vi "CRC32-CITT.vi"(8 "error in (no error)":errorcluster caption="错误输入（无错误）", 11 "Data":u8[](array[numeric]) format="%02x") -> (0 "error out":errorcluster caption="错误输出", 3 "CRC":u32 format="%08x")   [LabVIEW 2016]
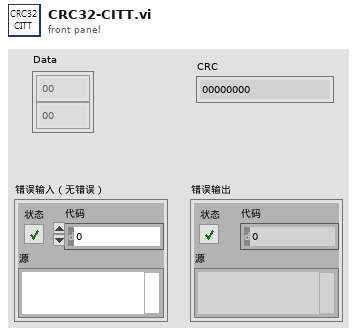
[diagram p1: front panel]
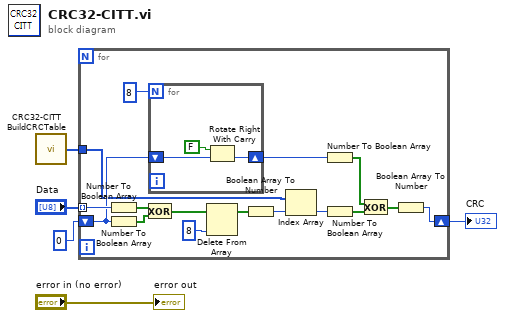
[diagram p0: block diagram]
diagram:
  n1 = call <userlib>:"CRC32-CITT BuildCRCTable.vi"() -> ("CRCTable"=w3:u32[])  [unwired: 5 in]
  n2 = for {
    tunnel: "Data" -> [w20] mode=indexing
    shift-right: [w7] -> w2
    shift-left: u32 0 -> [w19]
    tunnel: w3 -> [w13]
    n3 = Number To Boolean Array(number=w20) -> (Boolean array=w18:bool[])
    n4 = Number To Boolean Array(number=w19) -> (Boolean array=w17:bool[])
    n5 = Exclusive Or(1:w17, 2:w18) -> (0:w16:bool[])
    n6 = for {
      N: 8 -> [_]
      shift-right: [w22] -> w8
      shift-left: w19 -> [w24]
      n7 = Rotate Right With Carry(2:w24, 3:FALSE ("进位")) -> (0:w22:u32)  [unwired: 1 out]
    }
    n8 = Delete From Array(array=w16, index=8 ("索引")) -> (array with subset deleted=w14:bool[])  [unwired: 1 in, 1 out]
    n9 = Boolean Array To Number(Boolean array=w14) -> (number=w12:u32)
    n10 = Index Array(array=w13, index=w12) -> (element=w9:u32)
    n11 = Number To Boolean Array(number=w8) -> (Boolean array=w10:bool[])
    n12 = Number To Boolean Array(number=w9) -> (Boolean array=w11:bool[])
    n13 = Exclusive Or(1:w11, 2:w10) -> (0:w6:bool[])
    n14 = Boolean Array To Number(Boolean array=w6) -> (number=w7:u32)
  }
  "CRC" <- w2
  "error out" <- "error in (no error)"
